vi "Set.vi"(0 "Connection in":T1={"Baud"=9600, "Flow Ctl"=0, "COM port"="", "Parity"=0} {"Parity" items=["None", "Odd", "Even"]; "Flow Ctl" items=["None"]; "Baud" items=["4800"=4800, "9600"=9600, "19200"=19200, "38400"=38400]}, 1 "Variable":enum16{"Voltage", "Current"}(ring), 2 "Value":dbl, 3 "error in (no error)":errorcluster) -> (7 "Connection out":T1={"Baud"=9600, "Flow Ctl"=0, "COM port"="", "Parity"=0} {"Parity" items=["None", "Odd", "Even"]; "Flow Ctl" items=["None"]; "Baud" items=["4800"=4800, "9600"=9600, "19200"=19200, "38400"=38400]}, 8 "Actual Value":dbl, 10 "error out":errorcluster)   [LabVIEW 2014, in "B&K Precision 9120 series.lvclass"]
uses:
  B&K Precision 9120 series.lvclass
  Serial_Config.ctl
  <vilib>/Utility/error.llb/DialogType.ctl
  <vilib>/Utility/error.llb/Error Cluster From Error Code.vi
  <vilib>/ErrorRing/Error Ring.xnode
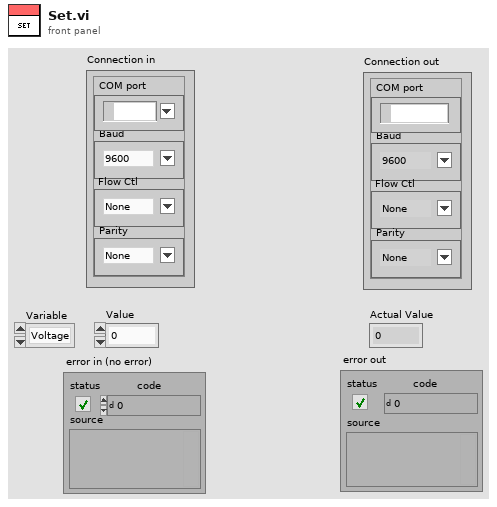
[diagram p1: front panel]
types:
  T1 = typedef "B&K Precision 9120 series.lvclass/Serial_Config.ctl" = cluster{"Baud":u32, "Flow Ctl":u16, "COM port":refnum<visa-resource-name>, "Parity":u16}
  T2 = typedef "DialogType.ctl" = u16
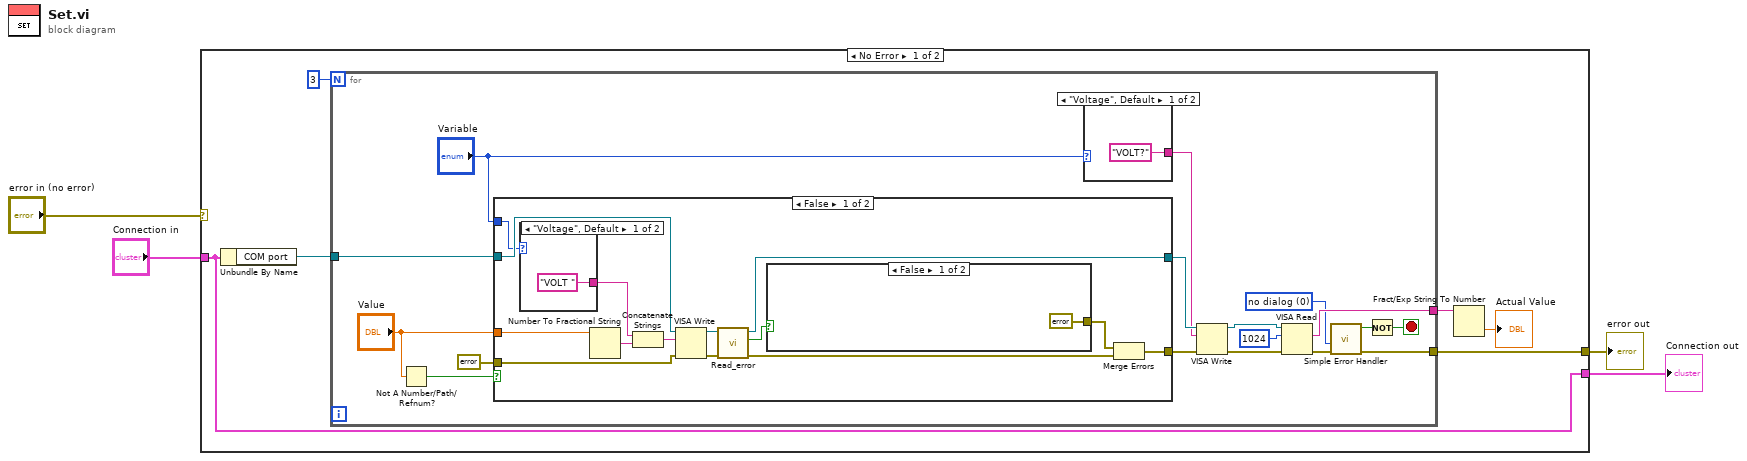
[diagram p0: block diagram]
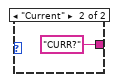
[diagram p2: hidden frame]
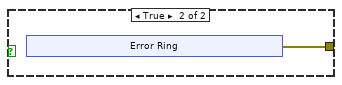
[diagram p3: hidden frame]
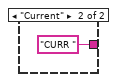
[diagram p4: hidden frame]
diagram:
  n1 = case shown="No Error" "error in (no error)" {
    selector: "error in (no error)" -> [_ w55]
    tunnel: [w7 w55] -> w4
    tunnel: "Connection in" -> [w5 w54]
    tunnel: [w5 w54] -> w1
    frame No Error {
      n2 = Unbundle By Name(w5) -> ("COM port"=w10:refnum<visa-resource-name>)
      n3 = for {
        N: 3 -> [_]
        tunnel: w10 -> [w27]
        tunnel: [w25] -> w9
        tunnel: [w15] -> w7
        stop <- w14 stop-if-true
        w16 = T2 0 items=["no dialog", "OK message", "continue or stop message", "OK message + warnings", "continue/stop + warnings"] ("type of dialog (OK msg:1)")
        n4 = Not A Number/Path/Refnum?(number/path/refnum="Value") -> (NaN/Path/Refnum?=w23:bool)
        n5 = case shown="False" w23 {
          tunnel: errorcluster {"status"=FALSE, "code"=0, "source"=""} ("error constant") -> [w43 w52]
          tunnel: w27 -> [w42 w53]
          tunnel: [w41 w53] -> w22
          tunnel: [w33 w52] -> w21
          tunnel: "Value" -> [w40 _]
          tunnel: "Variable" -> [w30 _]
          frame False {
            n6 = case shown="\"Voltage\", Default" w30 {
              tunnel: ["VOLT " ("write buffer") "CURR " ("write buffer")] -> w38
              frame "Voltage", Default {
              }
              frame "Current" {
              }
            }
            n7 = Number To Fractional String(number=w40) -> (F-format string=w37:string)  [unwired: 3 in]
            n8 = Concatenate Strings(w38, w37) -> (w39:string)
            n9 = VISA Write(VISA resource name=w42, write buffer=w39, error in (no error)=w43) -> (VISA resource name out=w36:refnum<visa-resource-name>, error out=w35:errorcluster)  [unwired: 1 out]
            n10 = call "Read_error.vi"("error in (no error)"=w35, "VISA resource in"=w36) -> ("error out"=w34:errorcluster, "Error"=w31:bool, "VISA resource out"=w41:refnum<visa-resource-name>)  [unwired: 7 in]
            n11 = case shown="False" w31 {
              tunnel: [errorcluster {"status"=FALSE, "code"=0, "source"=""} ("error constant") w45] -> w32
              frame False {
              }
              frame True {
                n12 = xnode "Error Ring"() -> ("error out"=w45:errorcluster)
              }
            }
            n13 = Merge Errors(w32, w34) -> (w33:errorcluster)
          }
          frame True {
          }
        }
        n14 = case shown="\"Voltage\", Default" "Variable" {
          tunnel: ["VOLT?" ("write buffer") "CURR?" ("write buffer")] -> w20
          frame "Voltage", Default {
          }
          frame "Current" {
          }
        }
        n15 = VISA Write(VISA resource name=w22, write buffer=w20, error in (no error)=w21) -> (VISA resource name out=w19:refnum<visa-resource-name>, error out=w18:errorcluster)  [unwired: 1 out]
        n16 = VISA Read(VISA resource name=w19, byte count=u32 1024, error in (no error)=w18) -> (read buffer=w25:string, error out=w17:errorcluster)  [unwired: 2 out]
        n17 = call <vilib>:"Simple Error Handler.vi"("type of dialog (OK msg:1)"=w16, "error in (no error)"=w17) -> ("error?"=w13:bool, "error out"=w15:errorcluster)  [unwired: 3 in, 3 out]
        n18 = Not(x=w13) -> (.not. x?=w14:bool)
      }
      n19 = Fract/Exp String To Number(string=w9) -> (number=→"Actual Value":dbl)  [unwired: 3 in, 1 out]
    }
    frame Error {
    }
  }
  "error out" <- w4
  "Connection out" <- w1
